vi "Temp (F) to Thermometer (C).vi"() -> ()   [LabVIEW 2017]
panel:
  out "F":dbl
  out "C":dbl
  in  "Temperature (F)":dbl(slide) scale=0.0..100.0
  out "Thermometer":dbl(slide) scale=0.0..100.0
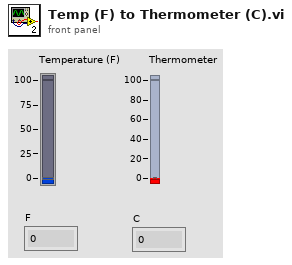
[diagram p1: front panel]
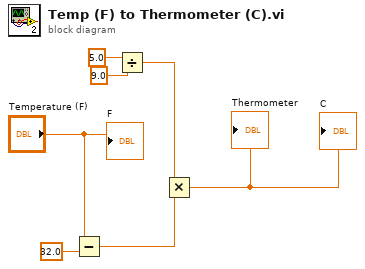
[diagram p0: block diagram]
diagram:
  n1 = Subtract(x="Temperature (F)", y=32.0) -> (x-y=w7:dbl)
  n2 = Divide(x=5.0, y=9.0) -> (x/y=w6:dbl)
  n3 = Multiply(x=w6, y=w7) -> (x*y=→"Thermometer" →"C":dbl)
  "F" <- "Temperature (F)"
